vi "Plateau.vi"(2 "Current for Gravity compensation":dbl, 3 "Position [deg] 3":dbl, 4 "Target Position [deg] 3":dbl) -> (0 "CurrentOut [A]":dbl, 1 "Boolean":bool)   [LabVIEW 2019]
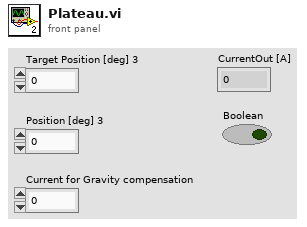
[diagram p1: front panel]
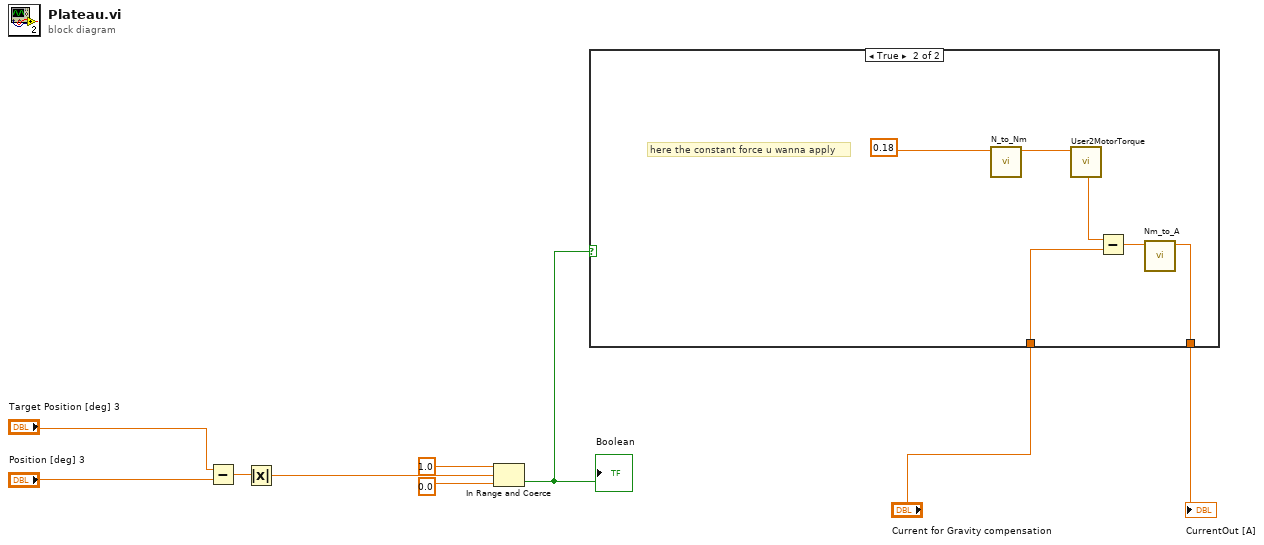
[diagram p0: block diagram]
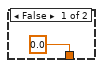
[diagram p2: hidden frame]
diagram:
  n1 = Subtract(x="Target Position [deg] 3", y="Position [deg] 3") -> (x-y=w4:dbl)
  n2 = Absolute Value(x=w4) -> (abs(x)=w5:dbl)
  n3 = In Range and Coerce(upper limit=1.0, x=w5, lower limit=0.0) -> (In Range?=w3:bool)  [unwired: 1 out]
  "Boolean" <- w3
  n4 = case shown="True" w3 {
    tunnel: [0.0 ("u") w15] -> w8
    tunnel: "Current for Gravity compensation" -> [_ w14]
    frame False {
    }
    frame True {
      # "here the constant force u wanna apply"
      n5 = call "N_to_Nm.vi"("Force [N]"=0.18) -> ("Torque [Nm]"=w16:dbl)  [unwired: 10 in]
      n6 = call "User2MotorTorque.vi"("User Torque [Nm]"=w16) -> ("Motor Torque [Nm]"=w12:dbl)  [unwired: 10 in]
      n7 = Subtract(x=w12, y=w14) -> (x-y=w13:dbl)
      n8 = call "Nm_to_A.vi"("Torque [Nm]"=w13) -> ("Current [A]"=w15:dbl)  [unwired: 10 in]
    }
  }
  "CurrentOut [A]" <- w8
